vi "classes.vi"(0 "HB_Factory.lvclass":refnum<class "HGF_DIMFactory.lvclass">, 1 "className":string, 5 "error in (no error)":errorcluster) -> (14 "HB_Factory.lvclass":refnum<class "HGF_DIMFactory.lvclass">, 16 "Object":refnum<class>, 19 "error out":errorcluster)   [LabVIEW 2012, in "HGF_DIM.lvlib" / "HGF_DIMFactory.lvclass"]
doc: "This dynamaic dispatch VI contains constant objects of all classes that can be produced by HGF_DIMFactory.\n\nChild classes can override it to define additional classes."
uses:
  HGF_DIMFactory.lvclass
  HGF_DIMCommand/HGF_DIMCommand.lvclass
  HGF_DIMEvent/HGF_DIMEvent.lvclass
  HGF_DIMService/HGF_DIMService.lvclass
  HGF_DIMSubscriber/HGF_DIMSubscriber.lvclass
  HGF_BaseClasses/HGF_Factory/HGF_Factory.lvclass
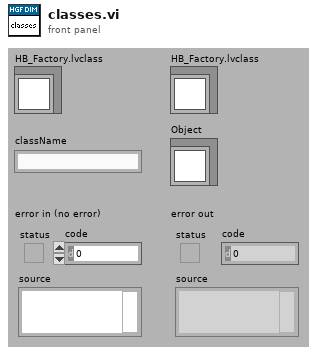
[diagram p1: front panel]
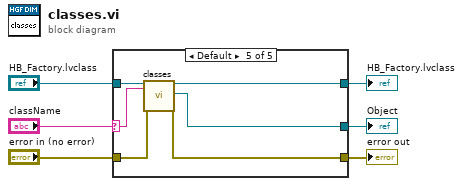
[diagram p0: block diagram]
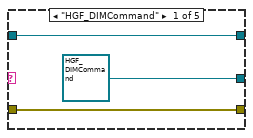
[diagram p2: hidden frame]
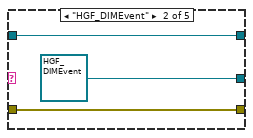
[diagram p3: hidden frame]
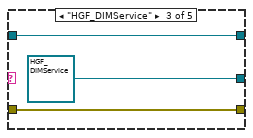
[diagram p4: hidden frame]
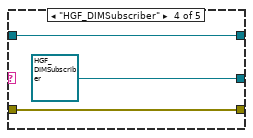
[diagram p5: hidden frame]
diagram:
  n1 = case shown="Default" "className" {
    selector: "className" -> [_ _ _ _ w19]
    tunnel: "HB_Factory.lvclass" -> [w9 w12 w15 w18 w24]
    tunnel: "error in (no error)" -> [w8 w11 w14 w17 w23]
    tunnel: [w9 w12 w15 w18 w22] -> w4
    tunnel: [refnum<class "HGF_DIMCommand.lvclass"> refnum ("HGF_DIM.lvlib:HGF_DIMCommand.lvclass") refnum<class "HGF_DIMEvent.lvclass"> refnum ("HGF_DIM.lvlib:HGF_DIMEvent.lvclass") refnum<class "HGF_DIMService.lvclass"> refnum ("HGF_DIM.lvlib:HGF_DIMService.lvclass") refnum<class "HGF_DIMSubscriber.lvclass"> refnum ("HGF_DIM.lvlib:HGF_DIMServiceSubscription.lvclass") w21] -> w3
    tunnel: [w8 w11 w14 w17 w20] -> w2
    frame "HGF_DIMCommand" {
    }
    frame "HGF_DIMEvent" {
    }
    frame "HGF_DIMService" {
    }
    frame "HGF_DIMSubscriber" {
    }
    frame Default {
      n2 = call-parent "classes.vi"("HGF_Factory"=w24, "className"=w19, "error in (no error)"=w23) -> ("HGF_Factory dup"=w22:refnum<class "HGF_DIMFactory.lvclass">, "Object"=w21:refnum<class>, "error out"=w20:errorcluster)  [unwired: 14 out]
    }
  }
  "error out" <- w2
  "HB_Factory.lvclass" <- w4
  "Object" <- w3
